vi "Memory.Pointer.Allocate.vi"(8 "error in (no error)":errorcluster, 10 "size":u64 format="%d bytes", 11 "Pointer in":refnum<class "Memory.Pointer.lvclass">) -> (0 "error out":errorcluster, 3 "Pointer out":refnum<class "Memory.Pointer.lvclass">)   [LabVIEW 2016, in "Memory.lvlib" / "Memory.Pointer.lvclass"]
uses:
  Memory.Pointer.lvclass
  Memory.Pointer.lvclass/Memory.Pointer.ctl
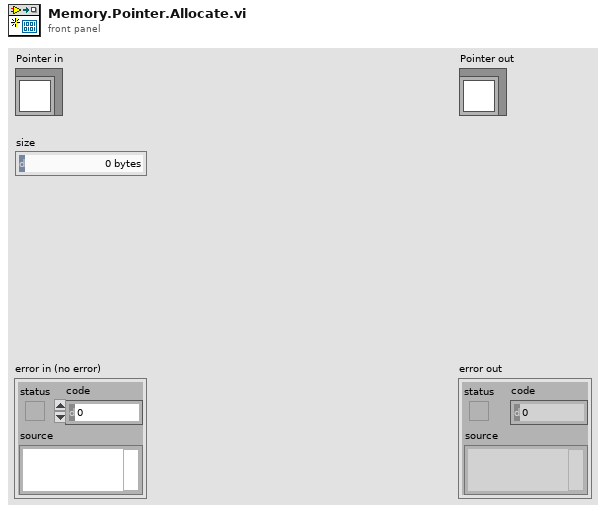
[diagram p1: front panel]
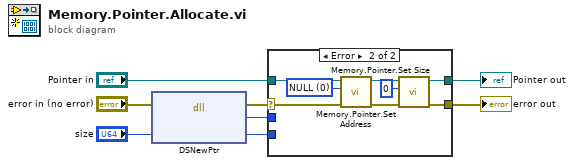
[diagram p0: block diagram]
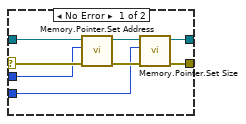
[diagram p2: hidden frame]
diagram:
  n1 = dll-call lib="LabVIEW" fn="DSNewPtr"(error in="error in (no error)", "size"="size") -> (error out=w6:errorcluster, "pointer"=w8:u64, "size"=w7:u64)  [unwired: 2 in, 1 out]
  n2 = case shown="Error" w6 {
    selector: w6 -> [w14 w16]
    tunnel: "Pointer in" -> [w13 w18]
    tunnel: w8 -> [w12 _]
    tunnel: [w10 w17] -> w5
    tunnel: w7 -> [w9 _]
    tunnel: [w14 w16] -> w3
    frame No Error {
      n3 = call "Memory.Pointer.Set Address.vi"("address"=w12, "Pointer in"=w13) -> ("Pointer out"=w11:refnum<class "Memory.Pointer.lvclass">)  [unwired: 9 in]
      n4 = call "Memory.Pointer.Set Size.vi"("size"=w9, "Pointer in"=w11) -> ("Pointer out"=w10:refnum<class "Memory.Pointer.lvclass">)  [unwired: 9 in]
    }
    frame Error {
      w15 = u64 0 items=["NULL"] ("Null")
      n5 = call "Memory.Pointer.Set Address.vi"("address"=w15, "Pointer in"=w18) -> ("Pointer out"=w19:refnum<class "Memory.Pointer.lvclass">)  [unwired: 9 in]
      n6 = call "Memory.Pointer.Set Size.vi"("size"=u64 0, "Pointer in"=w19) -> ("Pointer out"=w17:refnum<class "Memory.Pointer.lvclass">)  [unwired: 9 in]
    }
  }
  "error out" <- w3
  "Pointer out" <- w5
